vi "automated_scan_v1.1.vi"() -> ()   [LabVIEW 2018]
uses:
  Other_Libraries/MoCo Software/VI/global_m.vi
  <vilib>/Utility/file.llb/Write Delimited Spreadsheet (DBL).vi
  <vilib>/Utility/file.llb/Write Delimited Spreadsheet (string).vi
  Other_Libraries/Thorlabs_FW102C/Thorlabs_FW102C.lvlib
panel:
  out "End scan":errorcluster
  out "nloops":i32
  out "FW Position":i32
  out "Filter Wheel":errorcluster
  out "Current Wavelength(nm)":dbl
  out "Take Image":errorcluster
  out "Dark Integrating Time (s)":dbl caption="Elapsed Time (s)"
  out "% complete":dbl
  out "Total Steps":dbl
  in  "Tab Control":T1(tab)
  in  "Photodiode (VISA resource name)[Com3]":refnum<visa-resource-name>="COM3"
  in  "Mono port":refnum<visa-resource-name>="COM2"
  in  "Grating, gr/mm":u16(ring)=2 items=["2400", "1800", "1200", "600", "300", "150"]
  in  "Take Image":bool=TRUE
  in  "Two Cameras":bool=TRUE
  in  "Step Size":dbl=10.0
  in  "Stop Wavelength":dbl=600.0
  in  "Start Wavelength":dbl=500.0
  in  "Scan Directory":string="Peter_ferguson\\Tcal\\scans\\"
  in  "Scan Name":string="test_scan"
  in  "Scan Type":string(combo)="New Scan"
  in  "Photodiode / Camera\n Integration time(s)":dbl=10.0
  in  "Spectrometer Integration time":dbl=0.001
  out "VISA out":refnum<visa-resource-name>
  out "Current Value Bin":dbl format="%.6f"
  out "dup VISA session":refnum<visa-resource-name>
  out "dup VISA session 2":refnum<visa-resource-name>
  out "Mono wav":dbl format="%.3f"
  out "Photodiode 2":errorcluster
  out "Light Integrating Time (s)":dbl caption="Elapsed Time (s)"
  out "Active Wavelength":u32
  out "Serial Number":string
  out "Mono/Photodiode":errorcluster
  out "Step #":i32
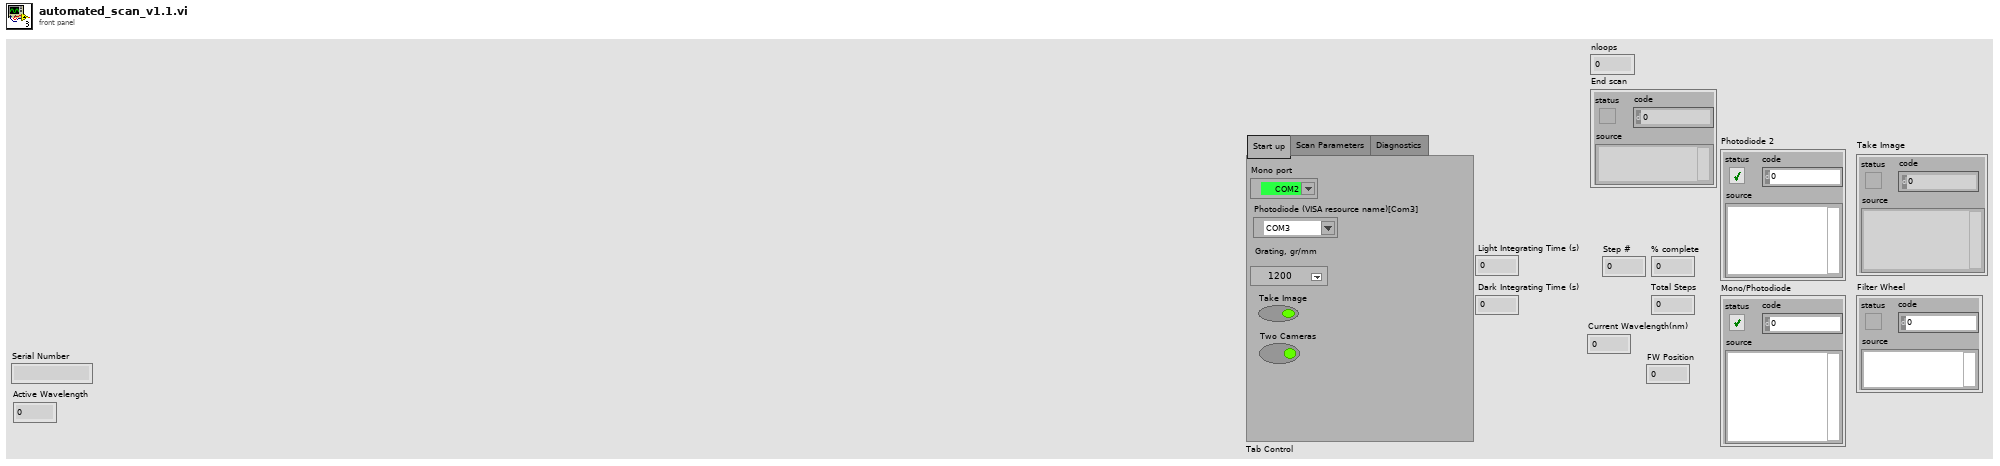
[diagram p1: front panel]
types:
  T1 = enum32{"Start up", "Scan Parameters", "Diagnostics"}
  T2 = cluster{"Head Type":u32, "Head Version":u32, "Serial Number":string, "Calibration Sensitivity":dbl, "Default Wavelength":u32, "Active Sensitivity":dbl, "Active Wavelength":u32, "Scale Min Power (Wattmeter)":u32, "Scale Max Power (Wattmeter)":u32, "Scale Min Energy":u32, "Scale Max Energy":u32, "Current Scale":u32, "Calo Mode":bool, "Anticipation":bool, "External Trig":bool, "Trig Level":dbl, "Zero Offset":dbl, "Multiplier 1":dbl, "Offset 1":dbl, "Multiplier 2":dbl, "Offset 2":dbl, "Max Power (Joulemeter)":dbl, "Max energy (Joulemeter)":dbl, "Currently Logging":bool, "Analog Out Active":bool, "Resolution":dbl, "Currently Calculating Stats":bool, "High-Resolution Display":bool, "Scale Min Wavelenght":u32, "Scale Max Wavelenght":u32, "Upper Bound":dbl, "Lower Bond":dbl, "Reference Value":dbl, "Thresholds Active":bool, "Fail":bool, "Attenuator":bool, "autoScale":bool, "IsdBm":bool}
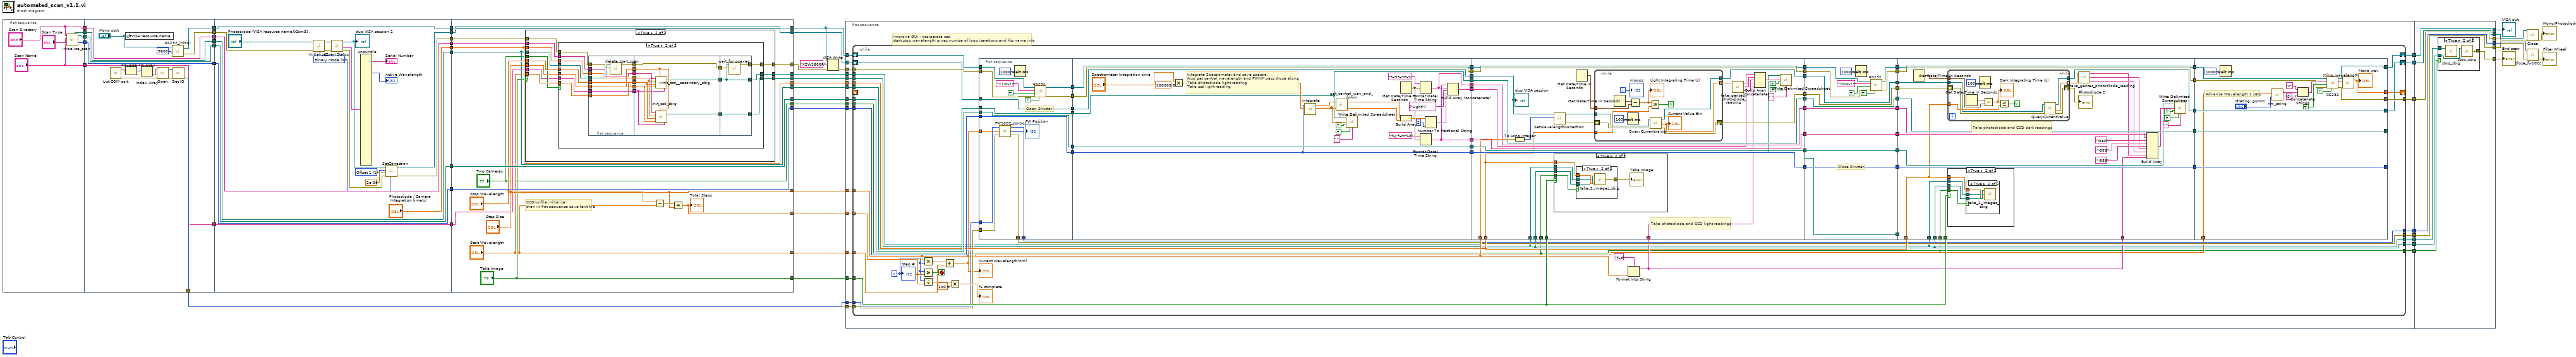
[diagram p0: block diagram]
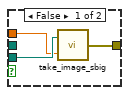
[diagram p3: hidden frame]
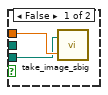
[diagram p5: hidden frame]
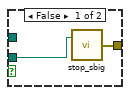
[diagram p6: hidden frame]
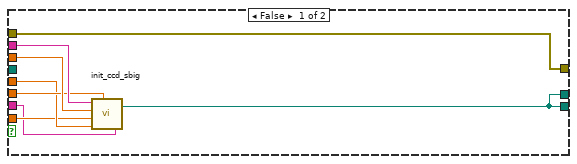
[diagram p8: hidden frame]
diagram:
  n1 = flat-sequence {
    tunnel: [w60] -> w43
    tunnel: [w59] -> w42
    tunnel: [w58] -> w41
    tunnel: ["Scan Directory"] -> w27
    tunnel: ["Scan Name"] -> w12
    tunnel: [w76] -> w40
    tunnel: [w75] -> w39
    tunnel: w43 -> [w74]
    tunnel: [w74] -> w38
    tunnel: w42 -> [w73]
    tunnel: [w73] -> w37
    tunnel: w41 -> [w72]
    tunnel: [w72] -> w36
    tunnel: w27 -> [w71]
    tunnel: [w71] -> w25
    tunnel: [w64] -> w19
    tunnel: [w63] -> w18
    tunnel: [w62] -> w13
    tunnel: w12 -> [w62]
    tunnel: w40 -> [w92]
    tunnel: [w92] -> w35
    tunnel: w39 -> [w88]
    tunnel: w38 -> [w91]
    tunnel: [w91] -> w34
    tunnel: w37 -> [w90]
    tunnel: [w90] -> w33
    tunnel: w36 -> [w89]
    tunnel: [w89] -> w32
    tunnel: [w85] -> w31
    tunnel: ["Photodiode / Camera\n Integration time(s)"] -> w30
    tunnel: [w81] -> w29
    tunnel: [w87] -> w26
    tunnel: w25 -> [w87]
    tunnel: [w79] -> w14
    tunnel: w13 -> [w79]
    tunnel: [w116] -> w45
    tunnel: w35 -> [w116]
    tunnel: [w107] -> w53
    tunnel: w34 -> [w107]
    tunnel: [w115] -> w52
    tunnel: w33 -> [w115]
    tunnel: [w114] -> w51
    tunnel: w32 -> [w114]
    tunnel: [w113] -> w50
    tunnel: w31 -> [w113]
    tunnel: [w111] -> w49
    tunnel: w30 -> [w111]
    tunnel: [w117] -> w44
    tunnel: w29 -> [w103]
    tunnel: [w102] -> w28
    tunnel: w26 -> [w112]
    tunnel: [w109] -> w24
    tunnel: ["Take Image"] -> w23
    tunnel: ["Step Size"] -> w21
    tunnel: ["Start Wavelength"] -> w20
    tunnel: w14 -> [w104]
    tunnel: [w101] -> w5
    tunnel: ["Two Cameras"] -> w4
    frame #0 {
      n2 = call "initialize_scan.vi"("Scan Directory"="Scan Directory", "Scan Name"="Scan Name", "Scan Type"="Scan Type") -> ("Path Spec"=w60:path, "Path Scan"=w58:path, "Wrapper Out"=w59:u64)  [unwired: 8 in, 2 out]
    }
    frame #1 {
      n3 = call "List COM port.vi"() -> ("error out"=w65:errorcluster, "COM Ports"=w68:string[])  [unwired: 10 in]
      n4 = global write "global_m.vi" "VISA resource name"("Mono port") -> ()
      n5 = Reverse 1D Array(array=w68) -> (reversed array=w67:string[])
      n6 = Index Array(array=w67) -> (element=w66:string)  [unwired: 1 in]
      n7 = call "Open.vi"("error in (no error)"=w65, "Serial Port"=w66) -> ("error out"=w69:errorcluster, "FW102C out"=w70:i32)  [unwired: 7 in, 1 out]
      n8 = call "RS232_initial.vi"("baud rate"=u32 9600, "VISA resource name"="Mono port") -> ("error out"=w75:errorcluster, "VISA name out"=w76:refnum<visa-resource-name>)  [unwired: 2 in]
      n9 = call "Get ID.vi"("error in (no error)"=w69, "FW102C in"=w70) -> ("error out"=w63:errorcluster, "FW102C out"=w64:i32)  [unwired: 7 in, 1 out]
    }
    frame #2 {
      w80 = u16 0 items=["Binary Mode", "Text Mode"] ("Transfer Type (binary)")
      w84 = u16 1 items=["Multiplier1", "Offset 1", "Multiplier 2", "Offset 2"] ("Correction Type")
      n10 = call "Initialize2.vi"("error in (no error)"=w88, "Instr. Descriptor (GPIB::)"="Photodiode (VISA resource name)[Com3]") -> ("error out"=w94:errorcluster, "VISA session"=w98:refnum<visa-resource-name>)  [unwired: 4 in]
      n11 = call "QueryStatus.vi"("error in (no error)"=w94, "VISA session"=w98) -> ("error out"=w82:errorcluster, "Status Data"=w97:T2, "dup VISA session"=w86:refnum<visa-resource-name>)  [unwired: 4 in, 1 out]
      "dup VISA session 2" <- w86
      n12 = Unbundle(w97) -> ("Serial Number"=→"Serial Number":string, "Active Wavelength"=→"Active Wavelength":u32)  [unwired: 36 out]
      n13 = call "SetCorrection.vi"("Transfer Type (binary)"=w80, "error in (no error)"=w82, "Correction  Value"=2e-09, "Correction Type"=w84, "VISA session"=w86) -> ("error out"=w81:errorcluster, "dup VISA session"=w85:refnum<visa-resource-name>)  [unwired: 3 in]
    }
    frame #3 {
      # "CCDrunfile initialize\nthen in flat sequence save text file"
      n14 = case shown="True" "Take Image" {
        tunnel: w112 -> [_ w132]
        tunnel: w111 -> [_ w131]
        tunnel: "Step Size" -> [_ w130]
        tunnel: "Stop Wavelength" -> [_ w129]
        tunnel: [w119 w128] -> w109
        tunnel: "Start Wavelength" -> [_ w127]
        tunnel: w107 -> [w119 w122]
        tunnel: "Two Cameras" -> [_ w126]
        tunnel: w104 -> [_ w125]
        tunnel: w103 -> [w120 w124]
        tunnel: [w120 w123] -> w102
        tunnel: [w119 w121] -> w101
        frame False {
        }
        frame True {
          n15 = case shown="True" w126 {
            tunnel: w132 -> [w140 w159]
            tunnel: w131 -> [w139 w158]
            tunnel: w130 -> [w138 w160]
            tunnel: w129 -> [w137 w156]
            tunnel: [w133 w161] -> w128
            tunnel: w127 -> [w136 w157]
            tunnel: w125 -> [w135 w155]
            tunnel: w124 -> [w134 w146]
            tunnel: [w134 w153] -> w123
            tunnel: w122 -> [_ w143]
            tunnel: [w133 w141] -> w121
            frame False {
              n16 = call "init_ccd_sbig.vi"("Scan Directory"=w140, "Exposure Time"=w139, "Min nm"=w136, "Max nm"=w137, "Step size"=w138, "Scan_prefix"=w135) -> ("Working Directory"=w133:path)
            }
            frame True {
              n17 = flat-sequence {
                tunnel: w155 -> [w165]
                tunnel: w156 -> [w166]
                tunnel: w157 -> [w167]
                tunnel: w158 -> [w168]
                tunnel: w159 -> [w169]
                tunnel: w160 -> [w170]
                tunnel: [w170] -> w152
                tunnel: [w169] -> w151
                tunnel: [w168] -> w150
                tunnel: [w167] -> w149
                tunnel: [w166] -> w148
                tunnel: [w165] -> w147
                tunnel: w146 -> [w164]
                tunnel: [w163] -> w144
                tunnel: w143 -> [w162]
                tunnel: [w173] -> w154
                tunnel: w152 -> [w179]
                tunnel: w151 -> [w178]
                tunnel: w150 -> [w177]
                tunnel: w149 -> [w176]
                tunnel: w148 -> [w175]
                tunnel: w147 -> [w174]
                tunnel: [w172] -> w145
                tunnel: w144 -> [w172]
                tunnel: [w171] -> w142
                tunnel: [w182] -> w161
                tunnel: w154 -> [w182]
                tunnel: [w183] -> w153
                tunnel: w145 -> [w181]
                tunnel: w142 -> [w180]
                tunnel: [w180] -> w141
                frame #0 {
                  n18 = call "delete_start_scan.vi"("error out"=w164, "base path"=w162) -> ("error out 2"=w163:errorcluster)  [unwired: 9 in]
                }
                frame #1 {
                  n19 = call "init_ccd__secondary_sbig.vi"("Scan Directory"=w178, "Exposure Time"=w177, "Min nm"=w176, "Max nm"=w175, "Step size"=w179, "Scan_prefix"=w174) -> ("Working Directory"=w171:path)
                  n20 = call "init_ccd_sbig.vi"("Scan Directory"=w178, "Exposure Time"=w177, "Min nm"=w176, "Max nm"=w175, "Step size"=w179, "Scan_prefix"=w174) -> ("Working Directory"=w173:path)
                }
                frame #2 {
                  n21 = call "wait_for_psexec.vi"("error out"=w181, "base path"=w180) -> ("error out 2"=w183:errorcluster)  [unwired: 9 in]
                }
              }
            }
          }
        }
      }
      n22 = Subtract(x="Stop Wavelength", y="Start Wavelength") -> (x-y=w118:dbl)
      n23 = Divide(x=w118, y="Step Size") -> (x/y=w117:dbl)
      "Total Steps" <- w117
    }
  }
  n24 = VISA Write(VISA resource name=w45, write buffer="X2W1600R", error in (no error)=w28) -> (error out=w54:errorcluster)  [unwired: 2 out]
  n25 = flat-sequence {
    tunnel: w54 -> [w207]
    tunnel: w53 -> [w206]
    tunnel: w52 -> [w205]
    tunnel: w51 -> [w204]
    tunnel: w50 -> [w203]
    tunnel: w49 -> [w202]
    tunnel: w45 -> [w199]
    tunnel: w44 -> [w198]
    tunnel: w24 -> [w197]
    tunnel: w23 -> [w196]
    tunnel: w21 -> [w194]
    tunnel: w20 -> [w193]
    tunnel: w19 -> [w192]
    tunnel: w18 -> [w191]
    tunnel: [w201] -> w11
    tunnel: [w200] -> w10
    tunnel: [w195] -> w9
    tunnel: [w190] -> w8
    tunnel: [w189] -> w7
    tunnel: [w188] -> w6
    tunnel: w5 -> [w187]
    tunnel: w4 -> [w186]
    tunnel: [w185] -> w2
    tunnel: [w184] -> w1
    tunnel: [w462] -> w15
    tunnel: [w463] -> w16
    tunnel: [w464] -> w22
    tunnel: [w465] -> w46
    tunnel: [w466] -> w48
    tunnel: w11 -> [w466]
    tunnel: w10 -> [w465]
    tunnel: w9 -> [w464]
    tunnel: w8 -> [w463]
    tunnel: w7 -> [w462]
    tunnel: w6 -> [w460]
    tunnel: [w461] -> w3
    tunnel: w2 -> [w459]
    tunnel: w1 -> [w458]
    frame #0 {
      # "Improve GUI, incorperate ccd,\nstart stop wavelength gives numbe of loop iterations and fits name info"
      n26 = while {
        tunnel: w207 -> [w277]
        tunnel: [w276] -> w201
        tunnel: w206 -> [w275]
        tunnel: w205 -> [w274]
        shift-right: [w228] -> _
        shift-left: _ -> [_]
        tunnel: w204 -> [w261]
        tunnel: w202 -> [w219]
        shift-right: [w229] -> w195
        shift-left: w203 -> [w251]
        shift-right: [w232] -> w200
        shift-left: w199 -> [w230]
        tunnel: w198 -> [w227]
        tunnel: w197 -> [w210]
        tunnel: w196 -> [w223]
        tunnel: w194 -> [w211]
        tunnel: w193 -> [w222]
        tunnel: w192 -> [w217]
        tunnel: w191 -> [w216]
        tunnel: [w214] -> w189
        tunnel: [w213] -> w190
        tunnel: [w210] -> w188
        tunnel: w187 -> [w209]
        tunnel: w186 -> [w208]
        tunnel: [w209] -> w185
        tunnel: [w208] -> w184
        i -> [w220]
        stop <- w240 stop-if-true
        n27 = Multiply(x=w211, y=w220) -> (x*y=w221:dbl)
        n28 = Greater Or Equal?(x=w220, y=w227) -> (x >= y?=w240:bool)
        n29 = Divide(x=w220, y=w227) -> (x/y=w226:dbl)
        n30 = Add(x=w221, y=w222) -> (x+y=w215:dbl)
        "Current Wavelength(nm)" <- w215
        n31 = Multiply(x=w226, y=100.0) -> (x*y=→"% complete":dbl)
        n32 = flat-sequence {
          tunnel: w277 -> [w294]
          tunnel: [w293] -> w273
          tunnel: [w292] -> w272
          tunnel: [w288] -> w271
          tunnel: w275 -> [w288]
          tunnel: w274 -> [w287]
          tunnel: [w287] -> w270
          tunnel: w261 -> [w286]
          tunnel: [w286] -> w260
          tunnel: w251 -> [w285]
          tunnel: [w285] -> w250
          tunnel: w230 -> [w284]
          tunnel: w217 -> [w283]
          tunnel: w216 -> [w282]
          tunnel: w215 -> [w281]
          tunnel: [w280] -> w214
          tunnel: [w279] -> w213
          tunnel: w273 -> [w321]
          tunnel: [w321] -> w259
          tunnel: w272 -> [w320]
          tunnel: [w320] -> w258
          tunnel: w271 -> [w312]
          tunnel: [w312] -> w257
          tunnel: w270 -> [w313]
          tunnel: [w313] -> w255
          tunnel: w260 -> [w301]
          tunnel: [w301] -> w253
          tunnel: [w300] -> w252
          tunnel: w250 -> [w299]
          tunnel: [w299] -> w249
          tunnel: [w297] -> w239
          tunnel: [w296] -> w234
          tunnel: w259 -> [w349]
          tunnel: w258 -> [w336]
          tunnel: w257 -> [w351]
          tunnel: [w351] -> w256
          tunnel: w255 -> [w350]
          tunnel: [w350] -> w254
          tunnel: w253 -> [w335]
          tunnel: w252 -> [w340]
          tunnel: w249 -> [w348]
          tunnel: [w349] -> w248
          tunnel: w219 -> [w328]
          tunnel: [w336] -> w247
          tunnel: [w335] -> w246
          tunnel: [w334] -> w244
          tunnel: [w333] -> w241
          tunnel: w239 -> [w332]
          tunnel: [w332] -> w238
          tunnel: [w331] -> w235
          tunnel: w234 -> [w331]
          tunnel: w210 -> [w329]
          tunnel: w223 -> [w327]
          tunnel: w212 -> [w324]
          tunnel: w215 -> [w326]
          tunnel: w209 -> [w323]
          tunnel: w208 -> [w322]
          tunnel: [w389] -> w269
          tunnel: [w388] -> w267
          tunnel: w256 -> [w384]
          tunnel: [w384] -> w265
          tunnel: [w383] -> w263
          tunnel: w254 -> [w383]
          tunnel: w248 -> [w382]
          tunnel: w247 -> [w381]
          tunnel: w246 -> [w376]
          tunnel: [w376] -> w245
          tunnel: w244 -> [w380]
          tunnel: [w380] -> w243
          tunnel: [w379] -> w242
          tunnel: w241 -> [w379]
          tunnel: w238 -> [w378]
          tunnel: [w378] -> w237
          tunnel: [w377] -> w236
          tunnel: w235 -> [w377]
          tunnel: [w376] -> w233
          tunnel: w269 -> [w419]
          tunnel: [w419] -> w268
          tunnel: w267 -> [w418]
          tunnel: [w418] -> w266
          tunnel: w265 -> [w417]
          tunnel: [w417] -> w264
          tunnel: w263 -> [w416]
          tunnel: [w416] -> w262
          tunnel: w245 -> [_]
          tunnel: w243 -> [w401]
          tunnel: w242 -> [w400]
          tunnel: w219 -> [w397]
          tunnel: w237 -> [w408]
          tunnel: w236 -> [w407]
          tunnel: w233 -> [w406]
          tunnel: [w399] -> w231
          tunnel: w210 -> [w396]
          tunnel: w223 -> [w395]
          tunnel: w212 -> [w393]
          tunnel: w209 -> [w392]
          tunnel: w208 -> [w391]
          tunnel: w268 -> [w454]
          tunnel: w266 -> [w455]
          tunnel: w264 -> [w444]
          tunnel: w262 -> [w446]
          tunnel: [w453] -> w232
          tunnel: [w452] -> w276
          tunnel: [w446] -> _
          tunnel: [w444] -> _
          tunnel: [w443] -> w229
          tunnel: w231 -> [w443]
          tunnel: [w442] -> w228
          tunnel: w211 -> [w441]
          frame #0 {
            # "Open Shutter"
            n33 = call "FW102C_control.vi"("error in (no error)"=w282, "Current Wavelength"=w281, "FW102C in"=w283) -> ("error out"=w279:errorcluster, "Position"=→"FW Position":i32, "FW102C out"=w280:i32)
            n34 = Wait (ms)(milliseconds to wait=u32 1000) -> ()  [unwired: 1 out]
            n35 = call "RS232.vi"("read"=TRUE, "error in"=w294, "write"=TRUE, "string to write"="Y1W-7?" ("string"), "VISA  name in"=w284) -> ("error out"=w292:errorcluster, "VISA out"=w293:refnum<visa-resource-name>)  [unwired: 1 in, 2 out]
          }
          frame #1 {
            # "Integrate Spectrometer and save spectra, \nAlso get central wavelength and FWHM pass those along\nTake photodiode light reading \nTake ccd light reading"
            n36 = Multiply(x="Spectrometer Integration time", y=100000.0) -> (x*y=w317:dbl)
            n37 = call "integrate.vi"("Numeric"=w317, "Wrapper Out"=w313) -> ("Spectrum Values"=w310:dbl[], "WL Values"=w311:dbl[])  [unwired: 7 in, 1 out]
            n38 = call "get_central_wav_and_fwhm.vi"("Signal"=w310, "Wavelenghs"=w311) -> ("FWHM"=w306:dbl, "Central"=w298:dbl)
            n39 = call-poly <vilib>:"Write Delimited Spreadsheet.vi"("file path (dialog if empty)"=w312, "1D data"=w310, "append to file? (new file:F)"=TRUE, "transpose? (no:F)"=FALSE, "delimiter (\\t)"="," ("delimiter (\\t)")) -> ()  [unwired: 9 in, 2 out]
            n40 = Get Date/Time In Seconds() -> (seconds since 1Jan1904=w308:timestamp)
            n41 = Build Array(w298, w306) -> (w305:dbl[])
            n42 = Format Date/Time String(time format string (%c)="%H%M%S", seconds (now)=w308) -> (date/time string=w296:string)  [unwired: 1 in]
            n43 = Format Date/Time String(time format string (%c)="%y%m%d", seconds (now)=w308) -> (date/time string=w297:string)  [unwired: 1 in]
            n44 = Number To Fractional String(number=w305, precision (6)=i16 2) -> (F-format string=w302:string[])  [unwired: 2 in]
            n45 = Build Array (concatenate)(w297, w296, string[] ["Light"] ("array"), w302) -> (w300:string[])
          }
          frame #2 {
            # "Take photodiode and CCD light readings"
            n46 = To Long Integer(number=w326) -> (32bit integer=w347:i32)
            n47 = call "SetWavelengthCorrection.vi"("Wave Length  ( 0= restore default)"=w347, "VISA session"=w348) -> ("error out"=w345:errorcluster, "dup VISA session"=w346:refnum<visa-resource-name>)  [unwired: 6 in]
            n48 = case shown="True" w327 {
              tunnel: w329 -> [_ w356]
              tunnel: w328 -> [_ w355]
              tunnel: w323 -> [_ w354]
              tunnel: w322 -> [_ w352]
              frame False {
              }
              frame True {
                n49 = case shown="True" w352 {
                  tunnel: w356 -> [w359 w362]
                  tunnel: w355 -> [w358 w363]
                  tunnel: w354 -> [_ w361]
                  tunnel: [w357 w360] -> w353
                  frame False {
                    n50 = call "take_image_sbig.vi"("Exptime"=w358, "path"=w359) -> ("error out"=w357:errorcluster)
                  }
                  frame True {
                    n51 = call "take_2_images_sbig.vi"("Exptime"=w363, "secondary path"=w361, "primary_path"=w362) -> ("error out"=w360:errorcluster)
                  }
                }
                "Take Image" <- w353
              }
            }
            n52 = Get Date/Time In Seconds() -> (seconds since 1Jan1904=w330:timestamp)
            n53 = while {
              tunnel: w346 -> [w375]
              shift-right: [w373] -> w333
              shift-left: w345 -> [w374]
              tunnel: w328 -> [w371]
              tunnel: [w370] -> w341 mode=indexing
              tunnel: [w369] -> w334
              tunnel: w330 -> [w367]
              i -> [w365]
              stop <- w372 continue-if-true
              n54 = Get Date/Time In Seconds() -> (seconds since 1Jan1904=w368:timestamp)
              n55 = Wait (ms)(milliseconds to wait=u32 100) -> ()  [unwired: 1 out]
              n56 = Subtract(x=w368, y=w367) -> (x-y=w366:dbl)
              "Light Integrating Time (s)" <- w366
              n57 = Less Or Equal?(x=w366, y=w371) -> (x <= y?=w372:bool)
              n58 = call "QueryCurrentValue.vi"("error in (no error)"=w374, "VISA session"=w375) -> ("error out"=w373:errorcluster, "Current Value Bin"=w370:dbl, "dup VISA session"=w369:refnum<visa-resource-name>)  [unwired: 3 in, 2 out]
              "Current Value Bin" <- w370
              "nloops" <- w365
            }
            n59 = call "take_gentec_photodiode_reading.vi"("numeric array"=w341) -> ("SD"=w338:string, "Mean"=w339:string, "Num of readings"=w325:string)  [unwired: 2 in]
            n60 = Build Array (concatenate)(w340, w339, w338, w325, w324) -> (w337:string[])
            n61 = call-poly <vilib>:"Write Delimited Spreadsheet.vi"("file path (dialog if empty)"=w335, "1D data"=w337, "append to file? (new file:F)"=TRUE, "transpose? (no:F)"=FALSE, "delimiter (\\t)"="," ("delimiter (\\t)")) -> ()  [unwired: 9 in, 2 out]
            "dup VISA session" <- w348
          }
          frame #3 {
            # "Close Shutter"
            n62 = Wait (ms)(milliseconds to wait=u32 1000) -> ()  [unwired: 1 out]
            n63 = call "RS232.vi"("read"=TRUE, "error in"=w381, "write"=TRUE, "string to write"="Y0W-7?" ("string"), "VISA  name in"=w382) -> ("error out"=w388:errorcluster, "VISA out"=w389:refnum<visa-resource-name>)  [unwired: 1 in, 2 out]
          }
          frame #4 {
            # "Take photodiode and CCD dark readings"
            n64 = Get Date/Time In Seconds() -> (seconds since 1Jan1904=w398:timestamp)
            n65 = while {
              shift-right: [w438] -> w411
              shift-left: w400 -> [w439]
              tunnel: [w436] -> w412 mode=indexing
              tunnel: w397 -> [w435]
              tunnel: w401 -> [w434]
              tunnel: [w433] -> w399
              tunnel: w398 -> [w431]
              stop <- w437 continue-if-true
              n66 = Get Date/Time In Seconds() -> (seconds since 1Jan1904=w432:timestamp)
              n67 = Wait (ms)(milliseconds to wait=u32 100) -> ()  [unwired: 1 out]
              n68 = Subtract(x=w432, y=w431) -> (x-y=w430:dbl)
              "Dark Integrating Time (s)" <- w430
              n69 = Less Or Equal?(x=w430, y=w435) -> (x <= y?=w437:bool)
              n70 = call "QueryCurrentValue.vi"("error in (no error)"=w439, "VISA session"=w434) -> ("error out"=w438:errorcluster, "Current Value Bin"=w436:dbl, "dup VISA session"=w433:refnum<visa-resource-name>)  [unwired: 3 in, 2 out]
            }
            "Photodiode 2" <- w411
            n71 = case shown="True" w395 {
              tunnel: w397 -> [_ w423]
              tunnel: w396 -> [_ w422]
              tunnel: w392 -> [_ w421]
              tunnel: w391 -> [_ w420]
              frame False {
              }
              frame True {
                n72 = case shown="True" w420 {
                  tunnel: w423 -> [w425 w427]
                  tunnel: w422 -> [w424 w428]
                  tunnel: w421 -> [_ w426]
                  frame False {
                    n73 = call "take_image_sbig.vi"("Exptime"=w425, "path"=w424) -> ()  [unwired: 1 out]
                  }
                  frame True {
                    n74 = call "take_2_images_sbig.vi"("Exptime"=w427, "secondary path"=w426, "primary_path"=w428) -> ()  [unwired: 1 out]
                  }
                }
              }
            }
            n75 = call "take_gentec_photodiode_reading.vi"("numeric array"=w412) -> ("SD"=w405:string, "Mean"=w404:string, "Num of readings"=w394:string)  [unwired: 2 in]
            n76 = Build Array(w408, w407, "Dark" ("date/time string"), "-999" ("element"), "-999" ("element"), w404, w405, w394, w393) -> (w409:string[])
            n77 = call-poly <vilib>:"Write Delimited Spreadsheet.vi"("file path (dialog if empty)"=w406, "1D data"=w409, "append to file? (new file:F)"=TRUE, "transpose? (no:F)"=FALSE, "delimiter (\\t)"="," ("delimiter (\\t)")) -> ()  [unwired: 9 in, 2 out]
          }
          frame #5 {
            # "Advance Wavelength 1 setp"
            n78 = Wait (ms)(milliseconds to wait=u32 1000) -> ()  [unwired: 1 out]
            n79 = call "nm_string.vi"("Grating, gr/mm"="Grating, gr/mm", "Wavelength, nm"=w441) -> ("nm_String"=w451:string)  [unwired: 2 in, 1 out]
            n80 = Concatenate Strings("X" ("string"), w451, "S" ("string")) -> (w448:string)
            n81 = call "RS232.vi"("read"=TRUE, "error in"=w455, "write"=TRUE, "string to write"=w448, "VISA  name in"=w454) -> ("error out"=w452:errorcluster, "read string"=w445:string, "VISA out"=w453:refnum<visa-resource-name>)  [unwired: 1 in, 1 out]
            n82 = call "string_wavelength.vi"("Position String"=w445) -> ("Present Wavelength"=w442:dbl)  [unwired: 3 in, 1 out]
            "Mono wav" <- w442
          }
        }
        n83 = Format Into String(format string="%d", w215) -> (resulting string=w212:string)  [unwired: 2 in, 1 out]
        "Step #" <- w220
      }
    }
    frame #1 {
      n84 = case shown="True" w458 {
        tunnel: [w468 w470] -> w461
        tunnel: w460 -> [w467 w471]
        tunnel: w459 -> [_ w469]
        frame False {
          n85 = call "stop_sbig.vi"("path"=w467) -> ("error out"=w468:errorcluster)  [unwired: 1 in]
        }
        frame True {
          n86 = call "stop_sbig.vi"("path"=w469) -> ()  [unwired: 1 in, 1 out]
          n87 = call "stop_sbig.vi"("path"=w471) -> ("error out"=w470:errorcluster)  [unwired: 1 in]
        }
      }
    }
  }
  n88 = call "Close.vi"("VISA session"=w22, "error in (no error)"=w48) -> ("error out"=→"Mono/Photodiode":errorcluster)  [unwired: 13 in]
  n89 = call "Close_fw102c.vi"("error in (no error)"=w16, "FW102C in"=w15) -> ("error out"=→"Filter Wheel":errorcluster)  [unwired: 9 in]
  "VISA out" <- w46
  "End scan" <- w3
